vi "RobotDistanciaPared.vi"() -> ()   [LabVIEW 2010]
uses:
  <vilib>/Platform/TimedLoop/XDataNode/XDataNode.xnode
  <vilib>/Platform/TimedLoop/XDataNode/timing_clust.ctl
  <vilib>/Platform/TimedLoop/XDataNode/nitl_modes.ctl
  <vilib>/Platform/TimedLoop/XDataNode/wakeup.ctl
  <vilib>/Instr/_visa.llb/VISA Configure Serial Port (Instr).vi
  <vilib>/Platform/TimedLoop/XDataNode/XDNodeRunTimeDep.lvlib
panel:
  in  "Min 2":dbl
  in  "Max 2":dbl
  in  "Min 1":dbl
  in  "Max 1":dbl
  out "String 2":string
  out "error out":errorcluster
  out "XY Graph":cluster{"Y":dbl[], "Y":dbl[]}[](graph)
  out "ang":u8
  out "String":string
  in  "Ajuste":dbl(slide) scale=0.0..10.0
  in  "Set Distancia":dbl(slide) scale=0.0..100.0
  in  "Buscar":bool
  in  "Automatico/Manual":bool
  out "Distancia":u8(slide) scale=0.0..300.0
  out "Distancia vs Tiempo":dynamicdata(graph)
  out "Atras 2":bool
  out "Adelante 2":bool
  in  "Direccion 2":bool
  in  "Velocidad 2":dbl(slide) scale=0.0..255.0
  out "Atras":bool
  out "Adelante":bool
  in  "Direccion":bool
  in  "Velocidad 1":dbl(slide) scale=0.0..255.0
  in  "Angulo Sensor Ultrasonico":dbl(knob) scale=0.0..160.0
  in  "Period                :":i64=1000
  in  "Flow control    :":u16(ring) items=["None"=0, "XON/XOFF"=1, "RTS/CTS"=2, "DTR/DSR"=4]
  in  "Stop bits         :":u16(ring)=10 items=["1.0"=10, "1.5"=15, "2.0"=20]
  in  "Paridad            :":u16(ring) items=["None", "Odd", "Even", "Mark", "Space"]
  in  "Data bits          :":u16=8 min=5 max=8 step=1
  in  "VISA resource : name:":refnum<visa-resource-name>="COM1"
  in  "Baud rate         :":u32=9600
  in  "stop":bool
  out "Read buffer":string
  out "var t":u8
  out "Manual":bool
  out "Auto":bool
  # "ROBOT MINI WALLE"
  # "Configuracion Serial"
  # "M\n1"
  # "M\n2"
  # "Hacia Derecha"
  # "Hacia Izquierda"
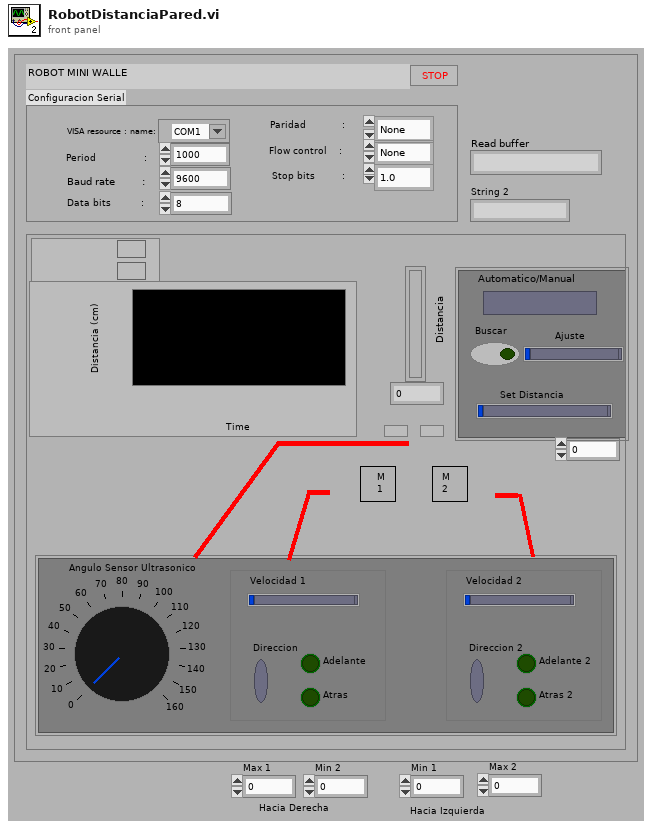
[diagram p1: front panel]
types:
  T1 = typedef "XDNodeRunTimeDep.lvlib/timing_clust.ctl" = cluster{"Expected End [f-1]":u64, "Actual End [f-1]":u64, "Finished Late? [f-1]":bool, "Expected End [i-1]":u64, "Actual End [i-1]":u64, "Finished Late? [i-1]":bool, "Expected Start [i]":u64, "Actual Start [i]":u64, "Expected Start [f]":u64, "Actual Start [f]":u64, "Source Name":string, "Structure Name":string, "Period":i64, "Deadline":i64, "Offset":i64, "Start":i64, "Priority":i32, "Timeout":i32, "Mode":T2, "Wakeup Reason":T3, "Error":errorcluster, "Source Type":string, "Secondary Source Type":string, "Global End Time":u64, "Global Start Time":u64, "Frame Duration":u64, "Iteration Duration":u64, "Assigned CPU":i32, "I/O Scan Engine Mode":u32}
  T2 = typedef "XDNodeRunTimeDep.lvlib/nitl_modes.ctl" = enum32{"No Change", "Process missed periods, maintain original phase", "Discard missed periods, maintain original phase", "Process missed periods, ignore original phase", "Discard missed periods, ignore original phase"}
  T3 = typedef "XDNodeRunTimeDep.lvlib/wakeup.ctl" = enum32{"Normal", "Aborted", "Asynchronous wakeup", "Timing source error", "Timed loop error", "Timeout"}
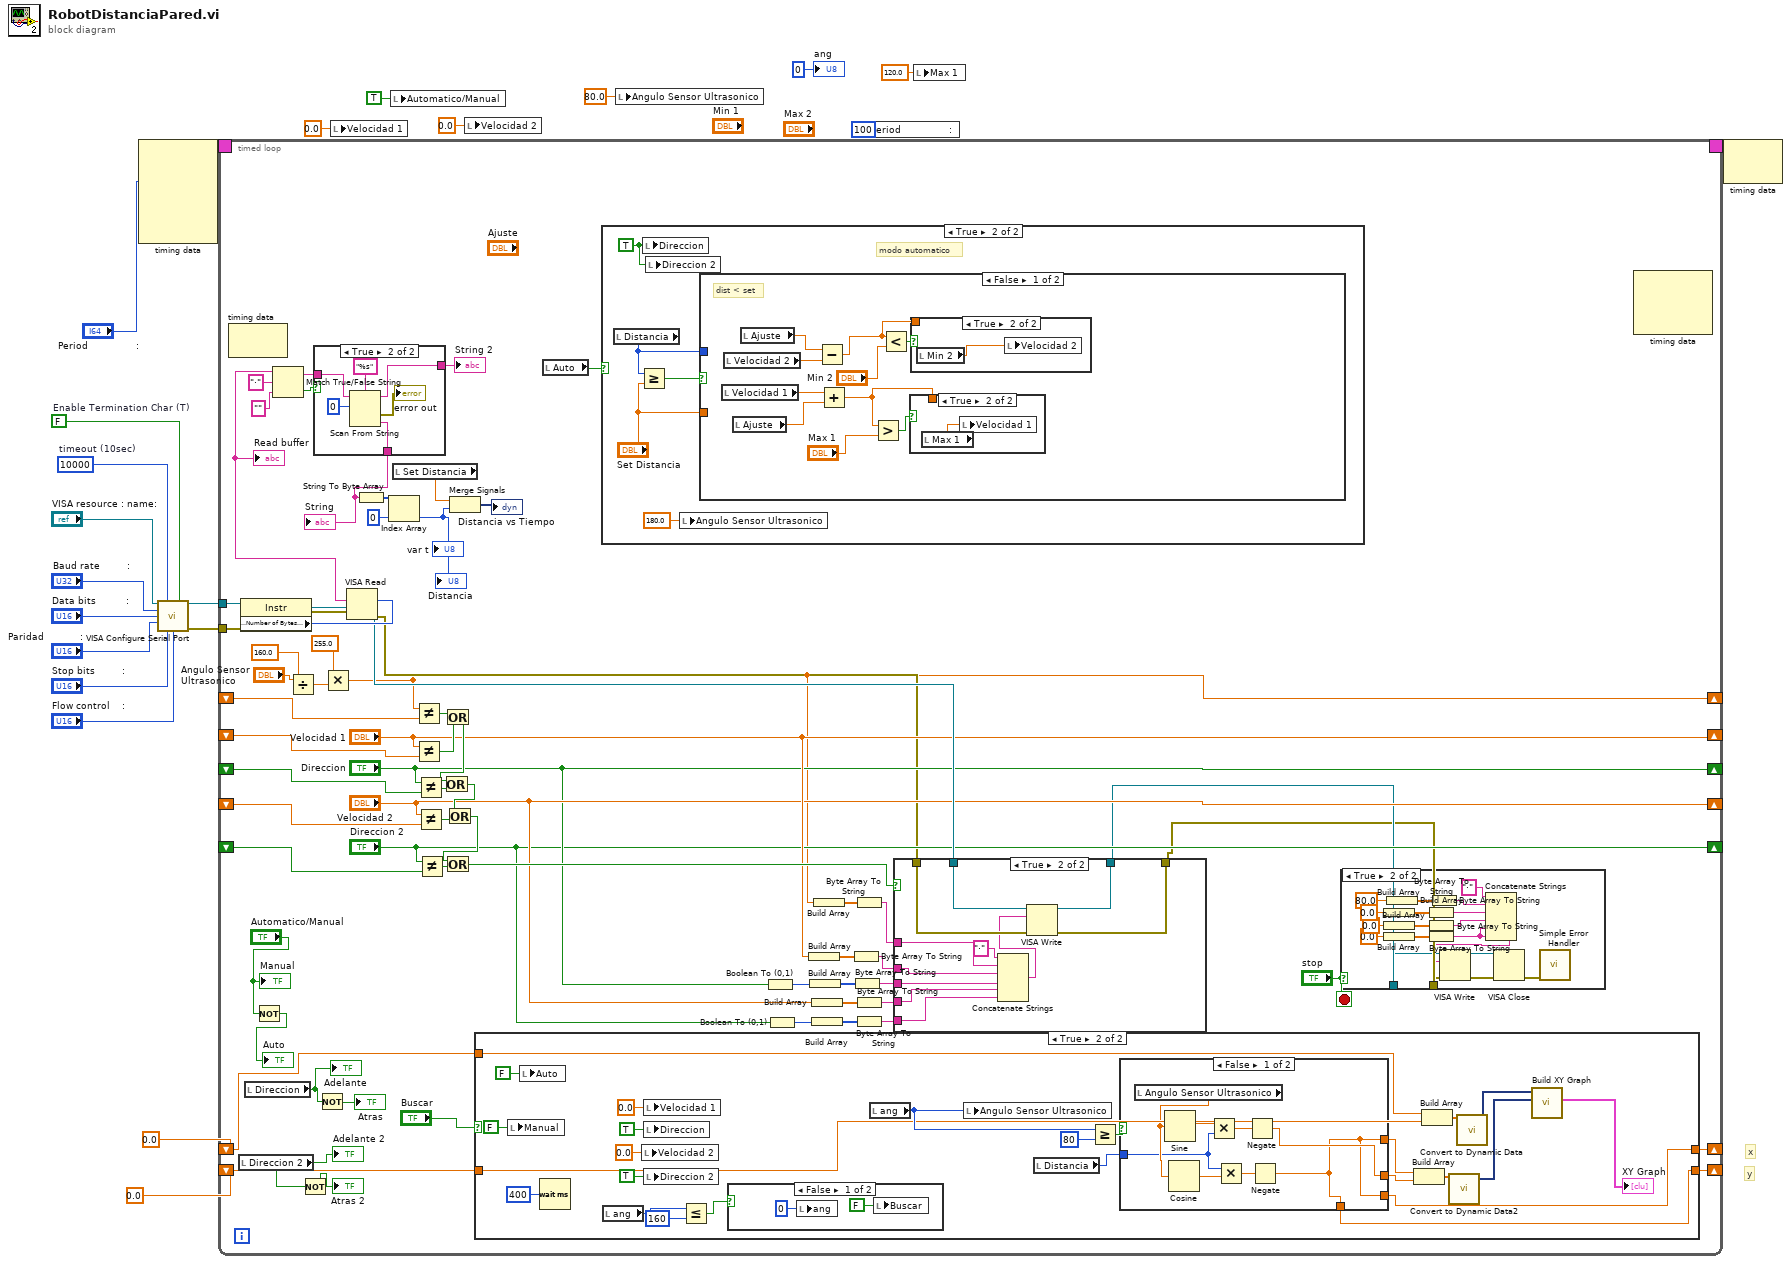
[diagram p0: block diagram]
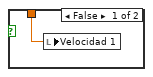
[diagram p3: hidden frame]
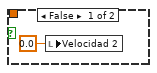
[diagram p4: hidden frame]
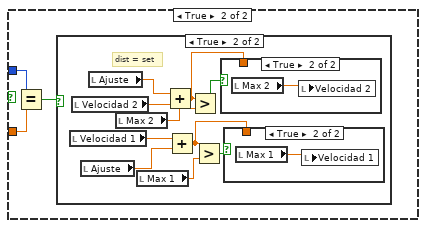
[diagram p5: hidden frame]
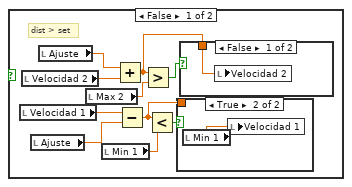
[diagram p6: hidden frame]
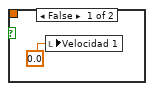
[diagram p7: hidden frame]
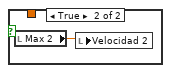
[diagram p8: hidden frame]
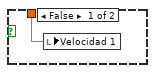
[diagram p9: hidden frame]
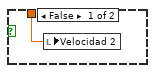
[diagram p10: hidden frame]
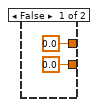
[diagram p11: hidden frame]
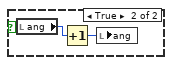
[diagram p12: hidden frame]
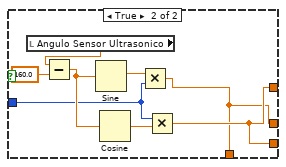
[diagram p13: hidden frame]
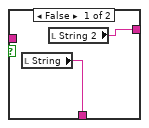
[diagram p15: hidden frame]
diagram:
  w16 = FALSE  # Enable Termination Char (T)
  w17 = u32 10000  # timeout (10sec)
  # "y"
  # "x"
  n1 = node-c288("Period                :") -> (w22:T1)  [unwired: 4 in]
  n2 = call-poly "VISA Configure Serial Port"("VISA resource name"="VISA resource : name:", "timeout (10sec)"=w17, "Enable Termination\nChar (T)"=w16, "baud rate (9600)"="Baud rate         :", "data bits (8)"="Data bits          :", "parity (0:none)"="Paridad            :", "stop bits (10: 1 bit)"="Stop bits         :", "flow control (0:none)"="Flow control    :") -> ("VISA resource name out"=w12:refnum<visa-resource-name>, "error out"=w11:errorcluster)  [unwired: 6 in]
  n3 = timed-loop {
    timing: w22 -> [_]
    timing-out: [_] -> w21
    tunnel: w12 -> [w84]
    tunnel: w11 -> [w83]
    shift-right: [w35] -> _
    shift-left: _ -> [w72]
    shift-right: ["Velocidad 1"] -> _
    shift-left: _ -> [w71]
    shift-right: ["Direccion"] -> _
    shift-left: _ -> [w70]
    shift-right: ["Velocidad 2"] -> _
    shift-left: _ -> [w69]
    shift-right: ["Direccion 2"] -> _
    shift-left: _ -> [w68]
    shift-right: [w31] -> _
    shift-left: 0.0 -> [w29]
    shift-right: [w30] -> _
    shift-left: 0.0 -> [w28]
    stop <- "stop" stop-if-true
    n4 = node-c288() -> ()  [unwired: 1 in, 1 out]
    n5 = local read "Direccion 2"() -> (w73:bool)
    "Adelante 2" <- w73
    n6 = property class="Instr"(reference=w84, error in=w83) -> (reference out=w85:refnum<visa-resource-name>, error out=w79:errorcluster, "Serial Settings:Number of Bytes at Serial Port"=w91:u32)
    n7 = local read "Direccion"() -> (w76:bool)
    "Adelante" <- w76
    n8 = Not(x="Automatico/Manual") -> (.not. x?=→"Auto":bool)
    n9 = Divide(x="Angulo Sensor Ultrasonico", y=160.0) -> (x/y=w37:dbl)
    n10 = Not(x=w73) -> (.not. x?=→"Atras 2":bool)
    n11 = Not(x=w76) -> (.not. x?=→"Atras":bool)
    n12 = Multiply(x=255.0, y=w37) -> (x*y=w35:dbl)
    n13 = VISA Read(VISA resource name=w85, byte count=w91, error in (no error)=w79) -> (VISA resource name out=w80:refnum<visa-resource-name>, read buffer=w89:string, error out=w44:errorcluster)  [unwired: 1 out]
    "Read buffer" <- w89
    n14 = Match True/False String(2:"" ("false string"), 3:"·" ("true string"), 4:w89) -> (0:w87:bool, 1:w40:string)
    n15 = case shown="True" w87 {
      tunnel: [w203 w207] -> w43
      tunnel: w40 -> [_ w206]
      tunnel: [w202 w204] -> w27
      frame False {
        n16 = local read "String"() -> (w203:string)
        n17 = local read "String 2"() -> (w202:string)
      }
      frame True {
        n18 = Scan From String(format string="%s", input string=w206, initial scan location=u32 0) -> (remaining string=w204:string, error out=→"error out":errorcluster, output 1=w207:string)  [unwired: 2 in, 1 out]
      }
    }
    "String" <- w43
    "String 2" <- w27
    n19 = String To Byte Array(string=w43) -> (unsigned byte array=w42:u8[])
    n20 = Index Array(array=w42, index=0) -> (element=w23:u8)
    "var t" <- w23
    "Distancia" <- w23
    n21 = local read "Set Distancia"() -> (w25:dbl)
    n22 = Not Equal?(x=w35, y=w72) -> (x != y?=w67:bool)
    n23 = Not Equal?(x="Velocidad 1", y=w71) -> (x != y?=w66:bool)
    n24 = Not Equal?(x="Direccion", y=w70) -> (x != y?=w64:bool)
    n25 = Not Equal?(x="Velocidad 2", y=w69) -> (x != y?=w63:bool)
    n26 = Not Equal?(x="Direccion 2", y=w68) -> (x != y?=w61:bool)
    n27 = Or(x=w67, y=w66) -> (x .or. y?=w65:bool)
    n28 = Or(x=w65, y=w64) -> (x .or. y?=w62:bool)
    n29 = Or(x=w62, y=w63) -> (x .or. y?=w60:bool)
    n30 = Or(x=w60, y=w61) -> (x .or. y?=w59:bool)
    n31 = Merge Signals(w25, w23) -> (→"Distancia vs Tiempo":dynamicdata)
    n32 = case shown="True" "Buscar" {
      tunnel: [0.0 w149] -> w31
      tunnel: [0.0 w148] -> w30
      tunnel: w29 -> [_ w145]
      tunnel: w28 -> [_ w144]
      frame False {
      }
      frame True {
        n33 = local write "Manual"(FALSE ("Manual")) -> ()
        n34 = local write "Auto"(FALSE ("Auto")) -> ()
        n35 = Wait (ms)(milliseconds to wait=u32 400) -> ()  [unwired: 1 out]
        n36 = local read "ang"() -> (w158:u8)
        n37 = local write "Velocidad 2"(0.0 ("Velocidad 2")) -> ()
        n38 = local write "Velocidad 1"(0.0 ("Velocidad 1")) -> ()
        n39 = local write "Direccion"(TRUE ("Direccion")) -> ()
        n40 = local write "Direccion 2"(TRUE ("Direccion 2")) -> ()
        n41 = Less Or Equal?(x=w158, y=u8 160) -> (x <= y?=w156:bool)
        n42 = case shown="False" w156 {
          frame False {
            n43 = local write "ang"(u8 0 ("ang")) -> ()
            n44 = local write "Buscar"(FALSE ("Buscar")) -> ()
          }
          frame True {
            n45 = local read "ang"() -> (w172:u8)
            n46 = Increment(x=w172) -> (x+1=w171:u8)
            n47 = local write "ang"(w171) -> ()
          }
        }
        n48 = local read "ang"() -> (w155:u8)
        n49 = local write "Angulo Sensor Ultrasonico"(w155) -> ()
        n50 = local read "Distancia"() -> (w159:u8)
        n51 = Greater Or Equal?(x=w155, y=80) -> (x >= y?=w161:bool)
        n52 = case shown="False" w161 {
          tunnel: w159 -> [w177 w183]
          tunnel: [w173 w182] -> w147
          tunnel: [w174 w181] -> w146
          tunnel: [w173 w182] -> w149
          tunnel: [w173 w181] -> w148
          frame False {
            n53 = local read "Angulo Sensor Ultrasonico"() -> (w178:dbl)
            n54 = Sine(x=w178) -> (sin(x)=w179:dbl)
            n55 = Cosine(x=w178) -> (cos(x)=w180:dbl)
            n56 = Multiply(x=w179, y=w177) -> (x*y=w176:dbl)
            n57 = Multiply(x=w177, y=w180) -> (x*y=w175:dbl)
            n58 = Negate(x=w176) -> (-x=w174:dbl)
            n59 = Negate(x=w175) -> (-x=w173:dbl)
          }
          frame True {
            n60 = local read "Angulo Sensor Ultrasonico"() -> (w188:dbl)
            n61 = Subtract(x=w188, y=160.0) -> (x-y=w186:dbl)
            n62 = Sine(x=w186) -> (sin(x)=w184:dbl)
            n63 = Cosine(x=w186) -> (cos(x)=w185:dbl)
            n64 = Multiply(x=w184, y=w183) -> (x*y=w181:dbl)
            n65 = Multiply(x=w183, y=w185) -> (x*y=w182:dbl)
          }
        }
        n66 = Build Array(w147, w146) -> (w150:dbl[])
        n67 = Build Array(w145, w144) -> (w151:dbl[])
        n68 = call "Convert to Dynamic Data2"("Array"=w150) -> ("Dynamic Data Type"=w152:dynamicdata)  [unwired: 3 in]
        n69 = call "Convert to Dynamic Data"("Array"=w151) -> ("Dynamic Data Type"=w153:dynamicdata)  [unwired: 3 in]
        n70 = call "Build XY Graph"("Y Input"=w152, "X Input"=w153) -> ("XY Graph"=→"XY Graph":cluster{"Y":dbl[], "Y":dbl[]}[])  [unwired: 3 in, 6 out]
      }
    }
    n71 = local read "Auto"() -> (w26:bool)
    n72 = case shown="True" w26 {
      frame False {
      }
      frame True {
        w95 = TRUE ("Direccion")
        # "modo automatico"
        n73 = local read "Distancia"() -> (w94:u8)
        n74 = Greater Or Equal?(x=w94, y="Set Distancia") -> (x >= y?=w96:bool)
        n75 = local write "Direccion"(w95) -> ()
        n76 = local write "Direccion 2"(w95) -> ()
        n77 = local write "Angulo Sensor Ultrasonico"(180.0 ("Angulo Sensor Ultrasonico")) -> ()
        n78 = case shown="False" w96 {
          tunnel: w94 -> [_ w113]
          tunnel: "Set Distancia" -> [_ w112]
          frame False {
            # "dist < set"
            n79 = local read "Velocidad 1"() -> (w103:dbl)
            n80 = local read "Velocidad 2"() -> (w106:dbl)
            n81 = local read "Ajuste"() -> (w104:dbl)
            n82 = local read "Ajuste"() -> (w105:dbl)
            n83 = Subtract(x=w105, y=w106) -> (x-y=w101:dbl)
            n84 = Add(x=w103, y=w104) -> (x+y=w99:dbl)
            n85 = Greater?(x=w99, y="Max 1") -> (0:w100:bool)
            n86 = Less?(x=w101, y="Min 2") -> (x < y?=w102:bool)
            n87 = case shown="True" w100 {
              tunnel: w99 -> [w107 _]
              frame False {
                n88 = local write "Velocidad 1"(w107) -> ()
              }
              frame True {
                n89 = local read "Max 1"() -> (w108:dbl)
                n90 = local write "Velocidad 1"(w108) -> ()
              }
            }
            n91 = case shown="True" w102 {
              tunnel: w101 -> [_ _]
              frame False {
                n92 = local write "Velocidad 2"(0.0 ("Velocidad 2")) -> ()
              }
              frame True {
                n93 = local read "Min 2"() -> (w110:dbl)
                n94 = local write "Velocidad 2"(w110) -> ()
              }
            }
          }
          frame True {
            n95 = Equal?(x=w113, y=w112) -> (x = y?=w111:bool)
            n96 = case shown="True" w111 {
              frame False {
                # "dist > set"
                n97 = local read "Velocidad 1"() -> (w120:dbl)
                n98 = local read "Velocidad 2"() -> (w123:dbl)
                n99 = local read "Ajuste"() -> (w121:dbl)
                n100 = local read "Ajuste"() -> (w122:dbl)
                n101 = local read "Max 2"() -> (w115:dbl)
                n102 = local read "Min 1"() -> (w114:dbl)
                n103 = Add(x=w122, y=w123) -> (x+y=w117:dbl)
                n104 = Subtract(x=w120, y=w121) -> (x-y=w116:dbl)
                n105 = Greater?(x=w117, y=w115) -> (0:w119:bool)
                n106 = Less?(x=w116, y=w114) -> (x < y?=w118:bool)
                n107 = case shown="True" w118 {
                  tunnel: w116 -> [_ _]
                  frame False {
                    n108 = local write "Velocidad 1"(0.0 ("Velocidad 1")) -> ()
                  }
                  frame True {
                    n109 = local read "Min 1"() -> (w125:dbl)
                    n110 = local write "Velocidad 1"(w125) -> ()
                  }
                }
                n111 = case shown="False" w119 {
                  tunnel: w117 -> [w126 _]
                  frame False {
                    n112 = local write "Velocidad 2"(w126) -> ()
                  }
                  frame True {
                    n113 = local read "Max 2"() -> (w127:dbl)
                    n114 = local write "Velocidad 2"(w127) -> ()
                  }
                }
              }
              frame True {
                # "dist = set"
                n115 = local read "Velocidad 1"() -> (w134:dbl)
                n116 = local read "Velocidad 2"() -> (w137:dbl)
                n117 = local read "Ajuste"() -> (w135:dbl)
                n118 = local read "Ajuste"() -> (w136:dbl)
                n119 = local read "Max 2"() -> (w129:dbl)
                n120 = local read "Max 1"() -> (w128:dbl)
                n121 = Add(x=w136, y=w137) -> (x+y=w130:dbl)
                n122 = Add(x=w134, y=w135) -> (x+y=w131:dbl)
                n123 = Greater?(x=w130, y=w129) -> (0:w133:bool)
                n124 = Greater?(x=w131, y=w128) -> (0:w132:bool)
                n125 = case shown="True" w133 {
                  tunnel: w130 -> [w140 _]
                  frame False {
                    n126 = local write "Velocidad 2"(w140) -> ()
                  }
                  frame True {
                    n127 = local read "Max 2"() -> (w141:dbl)
                    n128 = local write "Velocidad 2"(w141) -> ()
                  }
                }
                n129 = case shown="True" w132 {
                  tunnel: w131 -> [w138 _]
                  frame False {
                    n130 = local write "Velocidad 1"(w138) -> ()
                  }
                  frame True {
                    n131 = local read "Max 1"() -> (w139:dbl)
                    n132 = local write "Velocidad 1"(w139) -> ()
                  }
                }
              }
            }
          }
        }
      }
    }
    n133 = Boolean To (0,1)(Boolean="Direccion") -> (0, 1=w50:i16)
    n134 = Boolean To (0,1)(Boolean="Direccion 2") -> (0, 1=w48:i16)
    n135 = Build Array("Velocidad 1") -> (w57:dbl[])
    n136 = Build Array(w50) -> (w55:i16[])
    n137 = Build Array("Velocidad 2") -> (w54:dbl[])
    n138 = Build Array(w48) -> (w47:i16[])
    n139 = Build Array(w35) -> (w58:dbl[])
    n140 = Byte Array To String(unsigned byte array=w57) -> (string=w82:string)
    n141 = Byte Array To String(unsigned byte array=w55) -> (string=w53:string)
    n142 = Byte Array To String(unsigned byte array=w58) -> (string=w81:string)
    n143 = Byte Array To String(unsigned byte array=w54) -> (string=w52:string)
    n144 = Byte Array To String(unsigned byte array=w47) -> (string=w45:string)
    n145 = case shown="True" w59 {
      tunnel: w80 -> [w190 w201]
      tunnel: w44 -> [w189 w200]
      tunnel: [w190 w199] -> w33
      tunnel: [w189 w198] -> w32
      tunnel: w82 -> [_ w195]
      tunnel: w81 -> [_ w196]
      tunnel: w53 -> [_ w193]
      tunnel: w52 -> [_ w192]
      tunnel: w45 -> [_ w191]
      frame False {
      }
      frame True {
        n146 = Concatenate Strings("·" ("string"), w196, w195, w193, w192, w191) -> (w194:string)
        n147 = VISA Write(VISA resource name=w201, write buffer=w194, error in (no error)=w200) -> (VISA resource name out=w199:refnum<visa-resource-name>, error out=w198:errorcluster)  [unwired: 1 out]
      }
    }
    n148 = case shown="True" "stop" {
      tunnel: w33 -> [_ w225]
      tunnel: w32 -> [_ w224]
      frame False {
      }
      frame True {
        n149 = Build Array(0.0 ("element")) -> (w220:dbl[])
        n150 = Build Array(0.0 ("element")) -> (w219:dbl[])
        n151 = Build Array(0.0 ("element")) -> (w218:dbl[])
        n152 = Build Array(80.0 ("element")) -> (w221:dbl[])
        n153 = Byte Array To String(unsigned byte array=w220) -> (string=w212:string)
        n154 = Byte Array To String(unsigned byte array=w219) -> (string=w211:string)
        n155 = Byte Array To String(unsigned byte array=w218) -> (string=w210:string)
        n156 = Byte Array To String(unsigned byte array=w221) -> (string=w217:string)
        n157 = Concatenate Strings("·" ("string"), w217, w212, w211, w210, w210) -> (w222:string)
        n158 = VISA Write(VISA resource name=w225, write buffer=w222, error in (no error)=w224) -> (VISA resource name out=w227:refnum<visa-resource-name>, error out=w226:errorcluster)  [unwired: 1 out]
        n159 = VISA Close(VISA resource name=w227, error in (no error)=w226) -> (error out=w228:errorcluster)
        n160 = call <vilib>:"Simple Error Handler.vi"("error in (no error)"=w228) -> ()  [unwired: 4 in, 5 out]
      }
    }
    n161 = node-c288() -> ()  [unwired: 3 in, 1 out]
    "Manual" <- "Automatico/Manual"
  }
  n162 = local write "Velocidad 1"(0.0 ("Velocidad 1")) -> ()
  n163 = local write "Automatico/Manual"(TRUE ("Automatico/Manual")) -> ()
  n164 = local write "Velocidad 2"(0.0 ("Velocidad 2")) -> ()
  n165 = local write "Angulo Sensor Ultrasonico"(80.0 ("Angulo Sensor Ultrasonico")) -> ()
  n166 = local write "Period                :"(i64 100 ("Period")) -> ()
  n167 = local write "Max 1"(120.0 ("Max")) -> ()
  n168 = node-c288(w21) -> ()  [unwired: 1 out]
  "ang" <- u8 0 ("ang")
